vi "Init Response.vi"(8 "error in (no error)":errorcluster, 10 "Acquired Result.lvclass":refnum<class "Acquired Result.lvclass">, 11 "Measure Controller in":refnum<class "Measure Controller.lvclass">) -> (0 "error out":errorcluster, 3 "Measure Controller out":refnum<class "Measure Controller.lvclass">)   [LabVIEW 2015, in "Measure Controller.lvclass"]
uses:
  Measure Controller.lvclass
  Results/Acquired Result/Acquired Result.lvclass
  Measure Controller.lvclass/Measure Controller.ctl
  Measure Object/Measure Object.lvclass/Measure Object.ctl
  Measure Object/Read Reply to.vi
  Measure Object Messages/Result Reply Msg/Result Reply Msg.lvclass
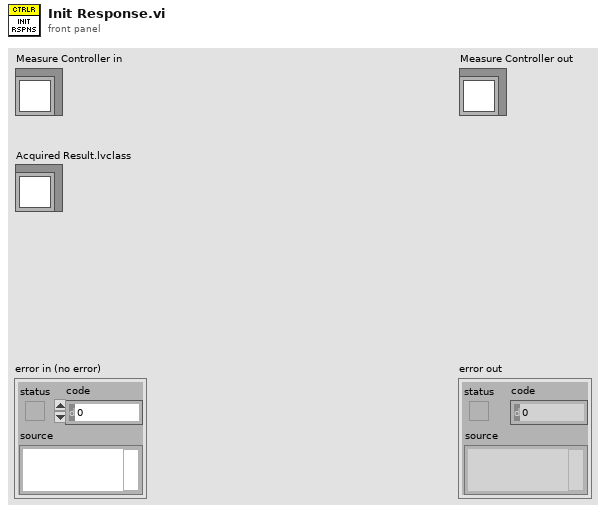
[diagram p1: front panel]
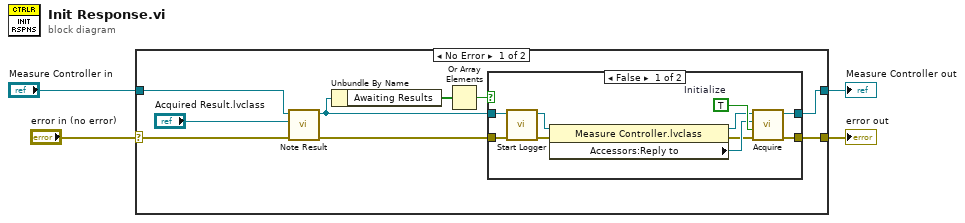
[diagram p0: block diagram]
diagram:
  n1 = case shown="No Error" "error in (no error)" {
    selector: "error in (no error)" -> [w12 w27]
    tunnel: [w5 w27] -> w3
    tunnel: [w7 w26] -> w1
    tunnel: "Measure Controller in" -> [w11 w26]
    frame No Error {
      n2 = call-dynamic "Note Result.vi"("error in (no error)"=w12, "Acquired Result.lvclass"="Acquired Result.lvclass", "Measure Controller in"=w11) -> ("error out"=w6:errorcluster, "Measure Controller out"=w8:refnum<class "Measure Controller.lvclass">)  [unwired: 7 in]
      n3 = Unbundle By Name(w8) -> ("Awaiting Results"=w10:bool[])
      n4 = Or Array Elements(Boolean array=w10) -> (logical OR=w9:bool)
      n5 = case shown="False" w9 {
        tunnel: w8 -> [w21 w25]
        tunnel: [w23 w25] -> w7
        tunnel: w6 -> [w20 w24]
        tunnel: [w22 w24] -> w5
        frame False {
          w19 = TRUE  # Initialize
          n6 = call-dynamic "Start Logger.vi"("error in (no error)"=w20, "Measure Controller in"=w21) -> ("error out"=w15:errorcluster, "Measure Controller out"=w18:refnum<class "Measure Controller.lvclass">)  [unwired: 7 in, 1 out]
          n7 = property class="Measure Controller.lvclass"(reference=w18, error in=w15) -> (reference out=w17:refnum<class "Measure Controller.lvclass">, error out=w14:errorcluster, "Accessors:Reply to"=w16:refnum<class "Result Reply Msg.lvclass">)
          n8 = call-dynamic "Acquire.vi"("error in (no error)"=w14, "Initialize"=w19, "Reply to"=w16, "Measure Controller in"=w17) -> ("error out"=w22:errorcluster, "Measure Controller out"=w23:refnum<class "Measure Controller.lvclass">)  [unwired: 6 in]
        }
        frame True {
        }
      }
    }
    frame Error {
    }
  }
  "error out" <- w3
  "Measure Controller out" <- w1
